vi "MethodToOverride.vi"(8 "error in (no error)":errorcluster, 11 "Level1Class in":refnum<class "Level1Class.lvclass">) -> (0 "error out":errorcluster, 3 "Level1Class out":refnum<class "Level1Class.lvclass">)   [LabVIEW 2019, in "Level1Class.lvlib" / "Level1Class.lvclass"]
uses:
  Level1Class.lvclass
  BaseClassDependency/BaseClassDependency.lvclass
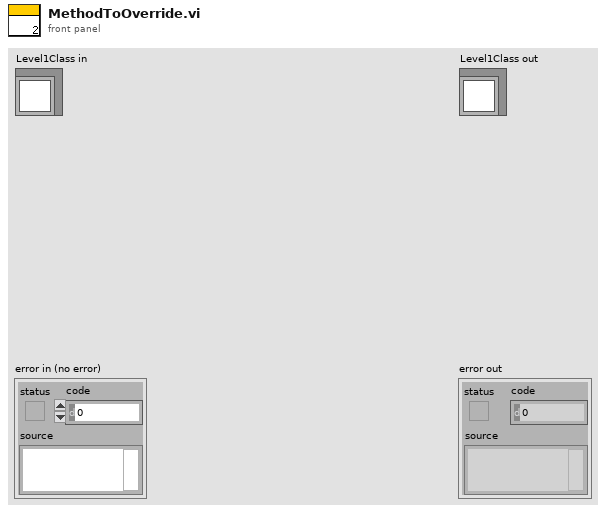
[diagram p1: front panel]
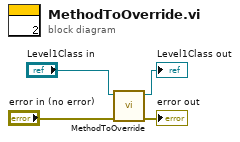
[diagram p0: block diagram]
diagram:
  n1 = call-parent "MethodToOverride.vi"("error in (no error)"="error in (no error)", "BaseClassDependency in"="Level1Class in") -> ("error out"=→"error out":errorcluster, "BaseClassDependency out"=→"Level1Class out":refnum<class "Level1Class.lvclass">)  [unwired: 8 in]
